vi "IsRefnum.vi"(8 "error in":errorcluster, 11 "SequenceRunReference in":refnum<class "SequenceRunReference.lvclass">) -> (0 "error out":errorcluster, 2 "IsRefnum":bool, 3 "SequenceRunReference out":refnum<class "SequenceRunReference.lvclass">)   [LabVIEW 2021, in "ProligentXMLGenerator.lvlib" / "SequenceRunReference.lvclass"]
doc: "Returns TRUE if the passed object is valid."
uses:
  SequenceRunReference.lvclass
  SequenceRunReference.lvclass/SequenceRunReference.ctl
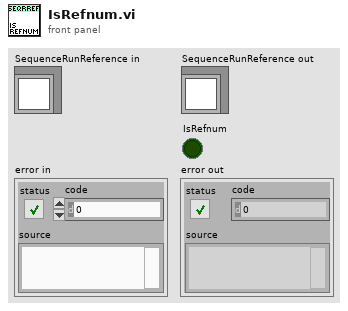
[diagram p1: front panel]
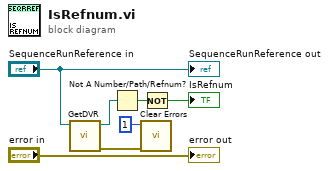
[diagram p0: block diagram]
diagram:
  n1 = call "GetDVR.vi"("SequenceRunReference in"="SequenceRunReference in") -> ("error out"=w1:errorcluster, "DVRReference"=w3:refnum<data-value>)  [unwired: 9 in]
  n2 = Not A Number/Path/Refnum?(number/path/refnum=w3) -> (NaN/Path/Refnum?=w5:bool)
  n3 = call <vilib>:"Clear Errors.vi"("error in (no error)"=w1, "specific error code to clear (0: all)"=1) -> ()  [unwired: 4 in, 2 out]
  n4 = Not(x=w5) -> (.not. x?=→"IsRefnum":bool)
  "error out" <- "error in"
  "SequenceRunReference out" <- "SequenceRunReference in"
